vi "FacadeResizable1DArray(I8).vi"(0 "Data In":T4, 2 "Display State In":T2, 3 "Container State":T3) -> (6 "Data Out":T4, 7 "Display State Out":T2, 8 "Action":T1)   [LabVIEW 2011, in "Resizable1DArray(I8).xctl"]
uses:
  <vilib>/_probes/SAPHIR/ViBox - Probes/Resizable1DArray/Resizable1DArray(I8)/Resizable1DArray(I8).xctl
  <vilib>/_probes/SAPHIR/ViBox - Probes/Resizable1DArray/Resizable1DArray(I8)/DataResizable1DArray(I8).ctl
  <vilib>/_xctls/Container State.ctl
  <vilib>/_probes/SAPHIR/ViBox - Probes/Resizable1DArray/Resizable1DArray(I8)/StateResizable1DArray(I8).ctl
  <vilib>/_xctls/Action.ctl
  <vilib>/_xctls/XControlSupport.lvlib
panel:
  in  "Format":string caption="Format :"
  out "Numeric":i8
  out "[I8]":i8[](array[numeric])
  # "Display Options"
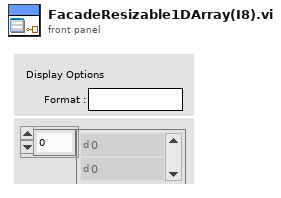
[diagram p1: front panel]
types:
  T1 = typedef "XControlSupport.lvlib/Action.ctl" = cluster{"Data Changed?":bool, "State Changed?":bool, "Action Name":string}
  T2 = typedef "Resizable1DArray(I8).xctl/StateResizable1DArray(I8).ctl" = cluster{"Height":u32}
  T3 = typedef "XControlSupport.lvlib/Container State.ctl" = cluster{"Indicator?":bool, "Run Mode?":bool, " Refnum":refnum<vi>}
  T4 = typedef "Resizable1DArray(I8).xctl/DataResizable1DArray(I8).ctl" = i8[]
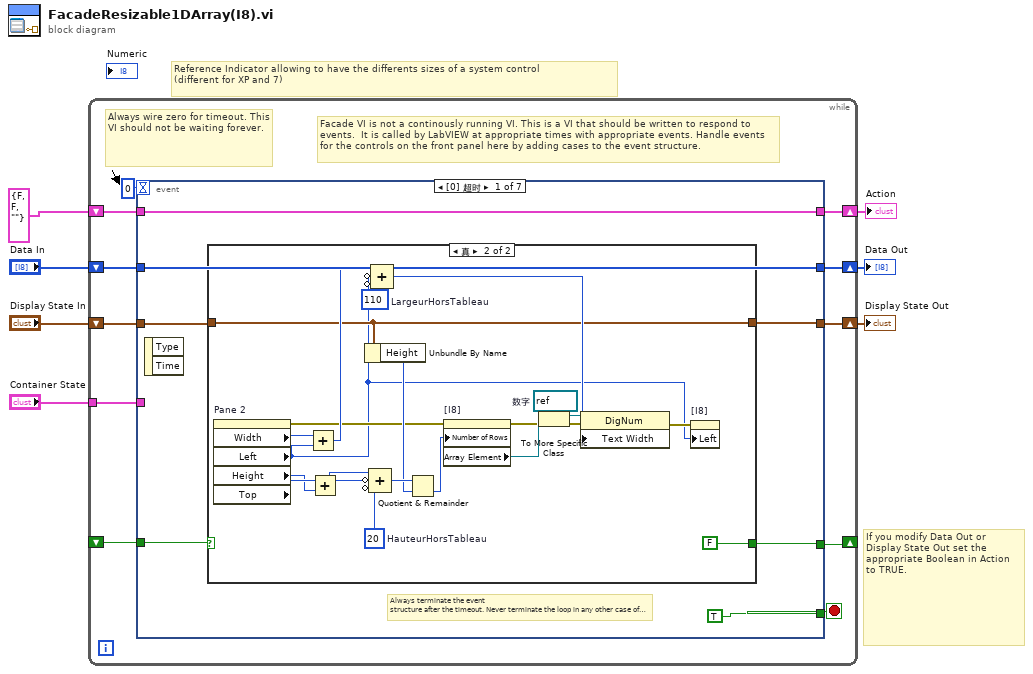
[diagram p0: block diagram]
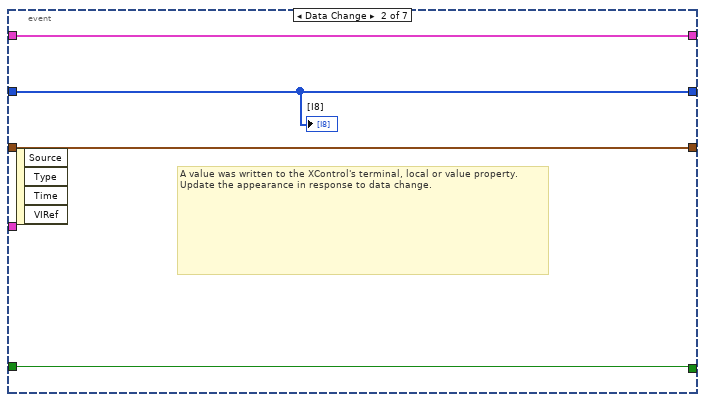
[diagram p3: hidden frame]
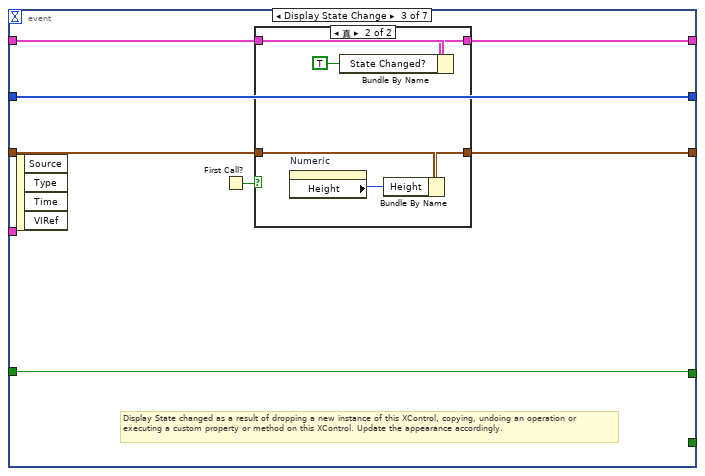
[diagram p4: hidden frame]
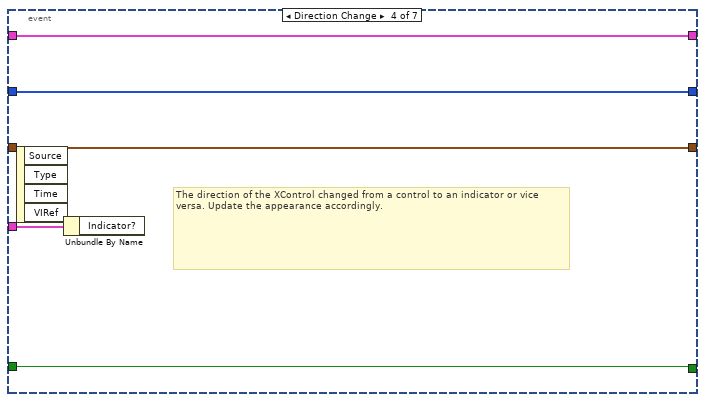
[diagram p6: hidden frame]
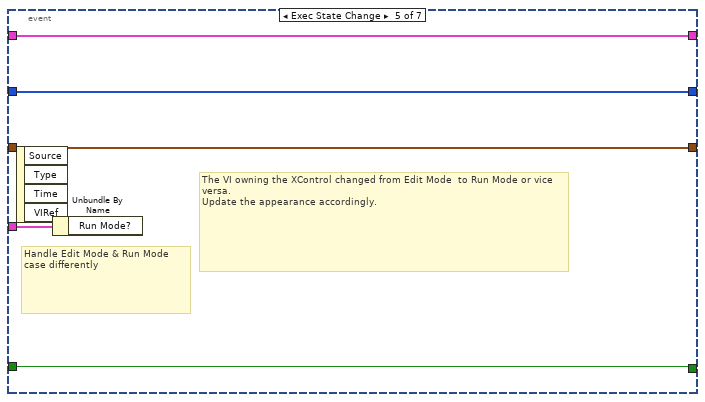
[diagram p7: hidden frame]
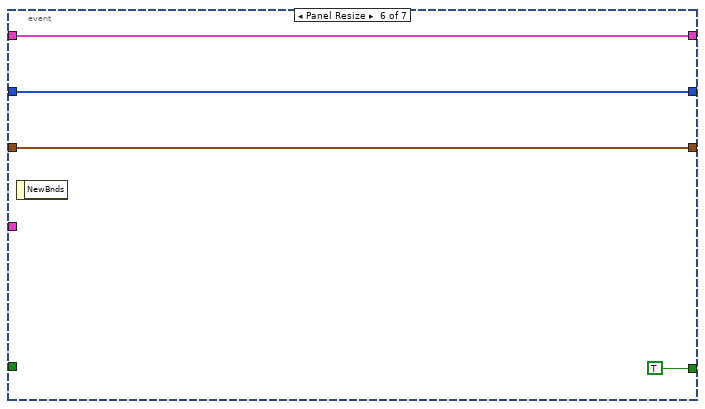
[diagram p8: hidden frame]
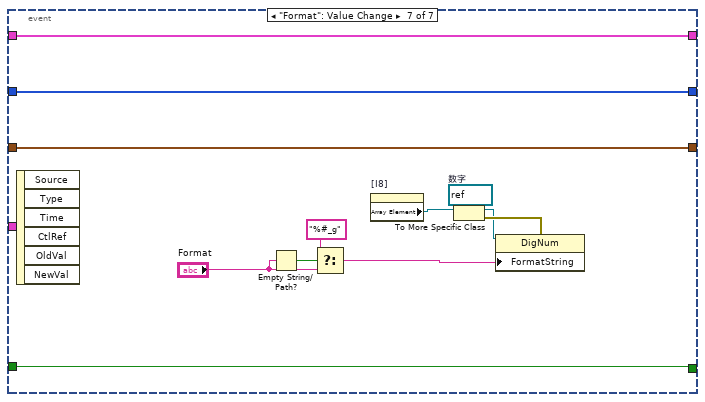
[diagram p9: hidden frame]
diagram:
  # "Reference Indicator allowing to have the differents sizes of a system control\n(different for XP and 7)"
  # "If you modify Data Out or\nDisplay State Out set the\nappropriate Boolean in Action\nto TRUE."
  n1 = while {
    shift-right: [w17] -> w5
    shift-left: "Display State In" -> [w18]
    tunnel: "Container State" -> [w14]
    shift-right: [w12] -> w7
    shift-left: "Data In" -> [w13]
    shift-right: [w10] -> w3
    shift-left: T1 {"Data Changed?"=FALSE, "State Changed?"=FALSE, "Action Name"=""} ("Action") -> [w11]
    shift-right: [w8] -> _
    shift-left: _ -> [w9]
    stop <- w16 stop-if-true
    # "Facade VI is not a continously running VI. This is a VI that should be written to respond to events.  It is called by LabVIEW at appropriate times with appropriate events. Handle events for the controls on the front panel here by adding cases to the event structure."
    # "Always wire zero for timeout. This\nVI should not be waiting forever."
    n2 = event shown="[0] 超时" {
      selector: _ -> [_ _ _ _ _ _ _]
      dyn-events: _ -> [_ _ _ _ _ _ _]
      timeout: 0 -> [_ _ _ _ _ _ _]
      tunnel: w18 -> [w20 w52 w54 w71 w76 w79 w90]
      tunnel: [w19 w52 w53 w71 w76 w79 w90] -> w17
      tunnel: [TRUE _ _ _ _ _ _] -> w16
      tunnel: w14 -> [_ _ _ w72 w77 _ _]
      tunnel: w13 -> [w23 w50 w59 w70 w75 w81 w91]
      tunnel: [w23 w50 w59 w70 w75 w81 w91] -> w12
      tunnel: [w24 w51 w55 w69 w74 w80 w92] -> w10
      tunnel: w11 -> [w24 w51 w56 w69 w74 w80 w92]
      tunnel: w9 -> [w22 w49 w58 w68 w73 _ w93]
      tunnel: [w21 w49 w58 w68 w73 TRUE w93] -> w8
      event Timeout {
        # "Always terminate the event\nstructure after the timeout. Never terminate the loop in any other case of the event structure."
        n3 = event-data() -> ()  [unwired: 3 out]
        n4 = case shown="真" w22 {
          selector: w22 -> [w27 _]
          tunnel: [w27 FALSE] -> w21
          tunnel: w20 -> [w26 w34]
          tunnel: [w26 w34] -> w19
          frame False {
          }
          frame True {
            w44 = refnum<vi> refnum  # 数字
            w46 = i16 20  # HauteurHorsTableau
            w45 = i16 110  # LargeurHorsTableau
            n5 = property on="Pane 2" class="Pane"() -> (error out=w32:errorcluster, "Width"=w29:u32, "Left"=w28:i32, "Height"=w30:u32, "Top"=w31:i32)  [unwired: 2 in, 1 out]
            n6 = Add(x=w29, y=w28) -> (x+y=w47:u32)
            n7 = Add(x=w31, y=w30) -> (x+y=w37:u32)
            n8 = Unbundle By Name(w34) -> ("Height"=w33:u32)
            n9 = Compound Arithmetic op=ADD(w37, invert w31, invert w46) -> (w41:u32)
            n10 = Compound Arithmetic op=ADD(w47, invert w28, invert w45) -> (w48:u32)
            n11 = Quotient & Remainder(x=w41, y=w33) -> (floor(x/y)=w36:u32)  [unwired: 1 out]
            n12 = property on="[I8]" class="Arr (严格)"(error in=w32, "Number of Rows"=w36) -> (error out=w40:errorcluster, "Array Element"=w42:refnum<vi>)  [unwired: 1 in, 1 out]
            n13 = To More Specific Class(target class=w44, reference=w42, error in=w40) -> (specific class reference=w43:refnum<vi>, error out=w39:errorcluster)
            n14 = property class="DigNum"(reference=w43, error in=w39, "Text Width"=w48) -> (error out=w38:errorcluster)  [unwired: 1 out]
            n15 = property on="[I8]" class="Arr (严格)"(error in=w38, "Left"=w28) -> ()  [unwired: 1 in, 2 out]
          }
        }
      }
      event Data Change {
        # "A value was written to the XControl's terminal, local or value property.\nUpdate the appearance in response to data change."
        n16 = event-data() -> ()  [unwired: 5 out]
        "[I8]" <- w50
      }
      event Display State Change {
        # "Display State changed as a result of dropping a new instance of this XControl, copying, undoing an operation or executing a custom property or method on this XControl. Update the appearance accordingly."
        n17 = event-data() -> ()  [unwired: 5 out]
        n18 = First Call?() -> (First Call?: T/F=w57:bool)
        n19 = case shown="真" w57 {
          tunnel: w54 -> [w61 w67]
          tunnel: [w61 w66] -> w53
          tunnel: w56 -> [w60 w64]
          tunnel: [w60 w63] -> w55
          frame False {
          }
          frame True {
            n20 = property on="Numeric" class="DigNum (严格)"() -> ("Height"=w65:u32)  [unwired: 2 in, 2 out]
            n21 = Bundle By Name(cluster=w64, "State Changed?"=TRUE) -> (w63:T1)
            n22 = Bundle By Name(cluster=w67, "Height"=w65) -> (w66:T2)
          }
        }
      }
      event Direction Change {
        # "The direction of the XControl changed from a control to an indicator or vice versa. Update the appearance accordingly."
        n23 = event-data() -> ()  [unwired: 5 out]
        n24 = Unbundle By Name(w72) -> ()  [unwired: 1 out]
      }
      event Exec State Change {
        # "The VI owning the XControl changed from Edit Mode  to Run Mode or vice versa.\nUpdate the appearance accordingly."
        # "Handle Edit Mode & Run Mode\ncase differently"
        n25 = event-data() -> ()  [unwired: 5 out]
        n26 = Unbundle By Name(w77) -> ()  [unwired: 1 out]
      }
      event Panel Resize {
        n27 = event-data() -> ()  [unwired: 2 out]
      }
      event "Format": Value Change {
        w83 = refnum<vi> refnum  # 数字
        n28 = event-data() -> ()  [unwired: 7 out]
        n29 = Empty String/Path?(string/path="Format") -> (empty?=w87:bool)
        n30 = Select(t="%#_g", s=w87, f="Format") -> (s? t:f=w89:string)
        n31 = property on="[I8]" class="Arr (严格)"() -> ("Array Element"=w86:refnum<vi>)  [unwired: 2 in, 2 out]
        n32 = To More Specific Class(target class=w83, reference=w86) -> (specific class reference=w84:refnum<vi>, error out=w85:errorcluster)  [unwired: 1 in]
        n33 = property class="DigNum"(reference=w84, error in=w85, "FormatString"=w89) -> ()  [unwired: 2 out]
      }
    }
  }
  "Display State Out" <- w5
  "Data Out" <- w7
  "Action" <- w3
